vi "ServiceShutdown.vi"(1 "In":i32) -> (0 "Out":i32)   [LabVIEW 2011]
doc: "Copyright (c) 2005, Kuan Chen\nAll rights reserved.\n\nRedistribution and use in source and binary forms, with or without modification, are permitted provided that the following conditions are met:\n\n * Redistributions of source code must retain the above copyright notice, this list of conditions and the following disclaimer.\n * Redistributions in binary form must reproduce the above copyright notice, this list of conditions and the following disclaimer in the documentation and/or other materials provided with the distribution.\n * Neither the name of the Kuan Chen nor the names of its contributors may be used to endorse or promote products derived from this software without specific prior written permission.\n\nTHIS SOFTWARE IS PROVIDED BY THE COPYRIGHT HOLDERS AND CONTRIBUTORS \"AS IS\" AND ANY EXPRESS OR IMPLIED WARRANTIES, INCLUDING, BUT NOT LIMITED TO, THE IMPLIED WARRANTIES OF MERCHANTABILITY AND FITNESS FOR A PARTICULAR PURPOSE ARE DISCLAIMED. IN NO EVENT SHALL THE COPYRIGHT OWNER OR CONTRIBUTORS BE LIABLE FOR ANY DIRECT, INDIRECT, INCIDENTAL, SPECIAL, EXEMPLARY, OR CONSEQUENTIAL DAMAGES (INCLUDING, BUT NOT LIMITED TO, PROCUREMENT OF SUBSTITUTE GOODS OR SERVICES; LOSS OF USE, DATA, OR PROFITS; OR BUSINESS INTERRUPTION) HOWEVER CAUSED AND ON ANY THEORY OF LIABILITY, WHETHER IN CONTRACT, STRICT LIABILITY, OR TORT (INCLUDING NEGLIGENCE OR OTHERWISE) ARISING IN ANY WAY OUT OF THE USE OF THIS SOFTWARE, EVEN IF ADVISED OF THE POSSIBILITY OF SUCH DAMAGE.\n\nStops the OutputThread.vi from continuing to output to the output file. Returns 0."
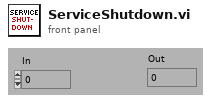
[diagram p1: front panel]
types:
  T1 = typedef "Rendezvous RefNum" = refnum<k1>
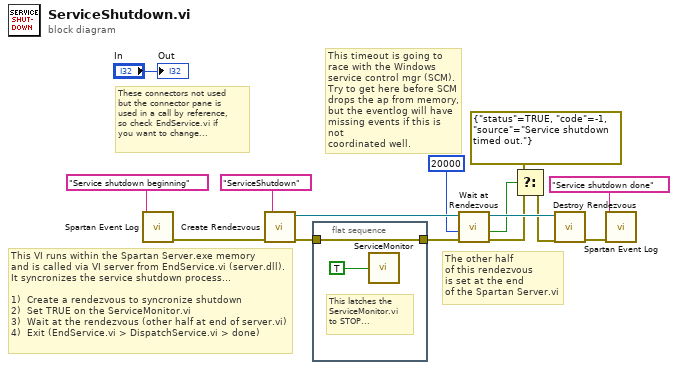
[diagram p0: block diagram]
diagram:
  # "The other half\nof this rendezvous\nis set at the end\nof the Spartan Server.vi"
  # "This timeout is going to\nrace with the Windows\nservice control mgr (SCM).\nTry to get here before SCM\ndrops the ap from memory,\nbut the eventlog will have\nmissing events if this is not\ncoordinated well."
  # "These connectors not used\nbut the connector pane is\nused in a call by reference,\nso check EndService.vi if\nyou want to change..."
  # "This VI runs within the Spartan Server.exe memory\nand is called via VI server from EndService.vi (server.dll).\nIt syncronizes the service shutdown process...\n\n1)  Create a rendezvous to syncronize shutdown\n2)  Set TRUE on the ServiceMonitor.vi\n3)  Wait at the rendezvous (other half at end of server.vi)\n4)  Exit (EndService.vi > DispatchService.vi > done)"
  n1 = call "Spartan Event Log.vi"("message (\"\")"="Service shutdown beginning" ("message (\"\")")) -> ("error out"=w11:errorcluster)  [unwired: 4 in, 3 out]
  n2 = call <vilib>:"Create Rendezvous.vi"("error in (no error)"=w11, "name (unnamed)"="ServiceShutdown" ("message (\"\")")) -> ("error out"=w9:errorcluster, "rendezvous"=w10:T1)  [unwired: 3 in, 1 out]
  n3 = flat-sequence {
    tunnel: w9 -> [w16]
    tunnel: [w16] -> w8
    frame #0 {
      # "This latches the\nServiceMonitor.vi\nto STOP..."
      n4 = call "ServiceMonitor.vi"("STOP"=TRUE) -> ()  [unwired: 1 out]
    }
  }
  n5 = call <vilib>:"Wait at Rendezvous.vi"("error in (no error)"=w8, "ms timeout (-1)"=20000, "rendezvous"=w10) -> ("error out"=w3:errorcluster, "timed out"=w4:bool, "rendezvous out"=w6:T1)  [unwired: 2 in]
  n6 = Select(t=errorcluster {"status"=TRUE, "code"=-1, "source"="Service shutdown timed out."}, s=w4, f=w3) -> (s? t:f=w2:errorcluster)
  n7 = call <vilib>:"Destroy Rendezvous.vi"("error in (no error)"=w2, "rendezvous"=w6) -> ("error out"=w5:errorcluster)  [unwired: 4 in, 1 out]
  n8 = call "Spartan Event Log.vi"("error in (no error)"=w5, "message (\"\")"="Service shutdown done" ("message (\"\")")) -> ()  [unwired: 3 in, 4 out]
  "Out" <- "In"
